vi "Allow_Access_Exchange_Tokens.vi"(7 "Client ID":string, 8 "error in (no error)":errorcluster, 11 "Location URL":string) -> (0 "error out":errorcluster, 1 "Authorization Code":string, 3 "body":string)   [LabVIEW 2016]
uses:
  Object Oriented Version/Response/Response.lvclass
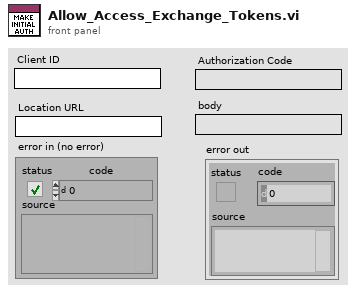
[diagram p1: front panel]
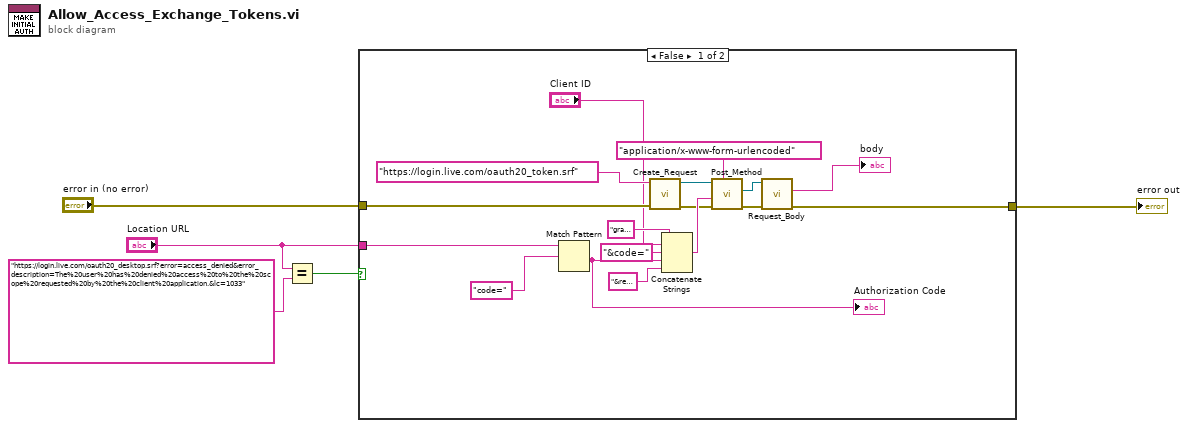
[diagram p0: block diagram]
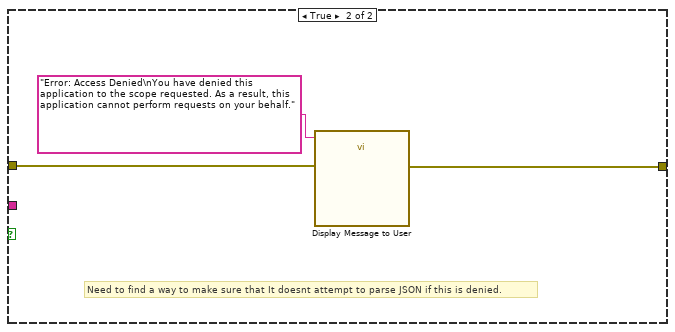
[diagram p2: hidden frame]
diagram:
  n1 = Equal?(x="Location URL", y="https://login.live.com/oauth20_desktop.srf?error=access_denied&error_description=The%20user%20has%20denied%20access%20to%20the%20scope%20requested%20by%20the%20client%20application.&lc=1033") -> (x = y?=w1:bool)
  n2 = case shown="False" w1 {
    tunnel: "error in (no error)" -> [w12 w25]
    tunnel: [w10 w24] -> w4
    tunnel: "Location URL" -> [w9 _]
    frame False {
      n3 = Match Pattern(string=w9, regular expression="code=") -> (after substring=w21:string)  [unwired: 1 in, 3 out]
      "Authorization Code" <- w21
      n4 = call "Create_Request.vi"("error in (no error)"=w12, "Base URL"="https://login.live.com/oauth20_token.srf" ("url")) -> ("error out"=w18:errorcluster, "Request out"=w19:refnum<class "Request.lvclass">)  [unwired: 8 in]
      n5 = Concatenate Strings("grant_type=authorization_code&client_id=", "Client ID", "&code=" ("string"), w21, "&redirect_uri=https://login.live.com/oauth20_desktop.srf") -> (w20:string)
      n6 = call "Post_Method.vi"("Body Content-Type"="application/x-www-form-urlencoded", "error in (no error)"=w18, "Body"=w20, "Request in"=w19) -> ("error out"=w17:errorcluster, "Response out"=w16:refnum<class "Response.lvclass">)  [unwired: 5 in, 1 out]
      n7 = call "Request_Body.vi"("error in (no error)"=w17, "Response in"=w16) -> ("error out"=w10:errorcluster, "Response Body"=→"body":string)  [unwired: 7 in, 1 out]
    }
    frame True {
      # "Need to find a way to make sure that It doesnt attempt to parse JSON if this is denied."
      n8 = call "Display Message to User"("error in (no error)"=w25, "Message"="Error: Access Denied\nYou have denied this application to the scope requested. As a result, this application cannot perform requests on your behalf.") -> ("error out"=w24:errorcluster)  [unwired: 8 in, 1 out]
    }
  }
  "error out" <- w4
